vi "readCommandApplyAOSCorrectionByForces.vi"(8 "error in (no error)":errorcluster, 10 "Parser":refnum<class "U8ArrayParserAutoIndexing.lvclass">, 11 "M1M3SAL in":refnum<class "M1M3SAL.lvclass">) -> (0 "error out":errorcluster, 2 "CommandApplyAOSCorrectionByForces":variant, 3 "M1M3SAL out":refnum<class "M1M3SAL.lvclass">)   [LabVIEW 2016, in "M1M3SupportCommunicator.lvlib" / "M1M3SAL.lvclass"]
uses:
  M1M3SAL.lvclass
  Common_RT_Utilities/U8ArrayParserAutoIndexing/U8ArrayParserAutoIndexing.lvclass
  DataTypes/Topics/CommandApplyAOSCorrectionByForces.ctl
  DataTypes/Topics/Parts/CommandId.ctl
  DataTypes/Topics/M1M3SupportTopics.lvlib
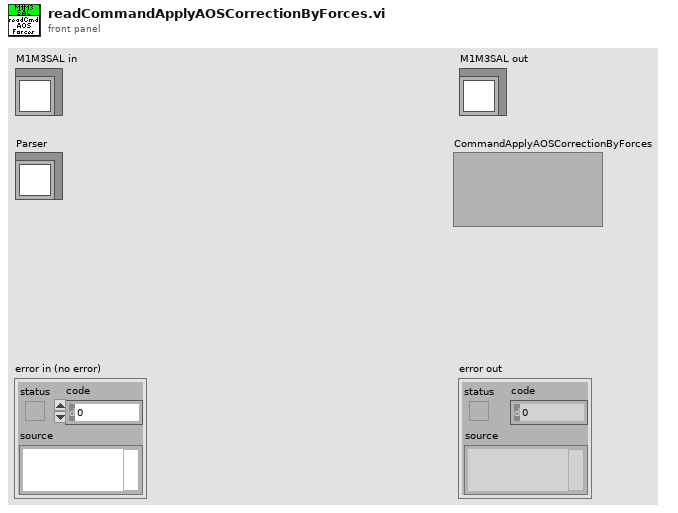
[diagram p1: front panel]
types:
  T1 = typedef "M1M3SupportTopics.lvlib/CommandApplyAOSCorrectionByForces.ctl" = cluster{"CommandId":T2, "ZForces":dbl[]}
  T2 = typedef "M1M3SupportTopics.lvlib/CommandId.ctl" = i32
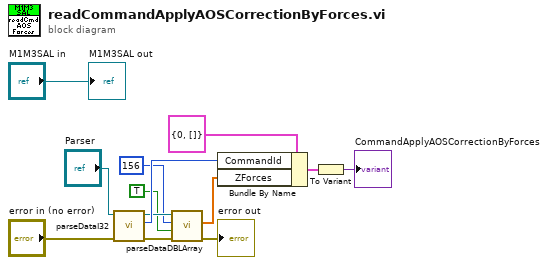
[diagram p0: block diagram]
diagram:
  n1 = call "parseDataI32.vi"("error in (no error)"="error in (no error)", "U8ArrayParserAutoIndexing in"="Parser") -> ("error out"=w6:errorcluster, "Data"=w8:i32, "U8ArrayParserAutoIndexing out"=w7:refnum<class "U8ArrayParserAutoIndexing.lvclass">)  [unwired: 7 in]
  n2 = call "parseDataDBLArray.vi"("U8ArrayParserAutoIndexing in"=w7, "Length"=156, "OverrideSwapBytes"=TRUE, "error in (no error)"=w6) -> ("Data"=w3:dbl[], "error out"=→"error out":errorcluster)  [unwired: 4 in, 1 out]
  n3 = Bundle By Name(cluster=T1 {"CommandId"=0, "ZForces"=[]} ("CommandApplyAOSCorrectionByForces"), "CommandId"=w8, "ZForces"=w3) -> (w12:T1)
  n4 = To Variant(anything=w12) -> (Variant=→"CommandApplyAOSCorrectionByForces":variant)
  "M1M3SAL out" <- "M1M3SAL in"
